vi "DT3120_ChopU16FromBArray.vi"(11 "BArray In":u8[](array[numeric])) -> (1 "Value":u16, 3 "BArray Out":u8[](array[numeric]))   [LabVIEW 8.6]
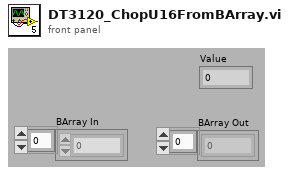
[diagram p1: front panel]
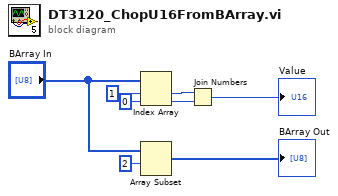
[diagram p0: block diagram]
diagram:
  n1 = Index Array(array="BArray In", index #1=1 ("index"), index #2=0 ("index")) -> (element #1=w6:u8, element #2=w7:u8)
  n2 = Array Subset(array="BArray In", index=2) -> (→"BArray Out":u8[])  [unwired: 1 in]
  n3 = Join Numbers(hi=w6, lo=w7) -> ((hi.lo)=→"Value":u16)
